vi "Spawn placeholder.vi"(11 "TEMPLATE Actor in":refnum<class "TEMPLATE Actor.lvclass">) -> (0 "Error out":errorcluster, 3 "TEMPLATE Actor out":refnum<class "TEMPLATE Actor.lvclass">)   [LabVIEW 2025, in "_Template.lvlib" / "Templates.lvlib" / "TEMPLATE Actor.lvlib" / "TEMPLATE Actor.lvclass"]
uses:
  TEMPLATE Actor.lvclass
  C:/git/jettl/src/jettl/jettl/Actor/Actor.lvclass
  Static Child UIDs.ctl
  TEMPLATE Actor.lvclass/TEMPLATE Actor.ctl
  C:/git/jettl/src/jettl Tools/_Template/Templates/TEMPLATE Actor/TEMPLATE Actor/TEMPLATE Actor.lvclass
  jettl/jettl/jettl.lvlib
  TEMPLATE Actor.lvlib
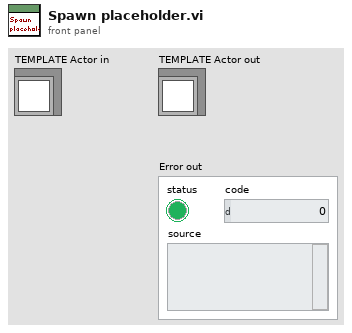
[diagram p1: front panel]
types:
  T1 = typedef "_Template.lvlib/Templates.lvlib/TEMPLATE Actor.lvlib/TEMPLATE Actor.lvclass/Static Child UIDs.ctl" = enum16{"placeholder"}
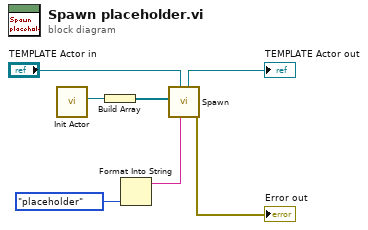
[diagram p0: block diagram]
diagram:
  n1 = call "Init Actor.vi"() -> ("Actor"=w3:refnum<class "Actor.lvclass">)  [unwired: 11 in]
  n2 = Build Array(w3) -> (w2:refnum<class "Actor.lvclass">[])
  n3 = Format Into String(Static_Child_UIDs."placeholder" ("Static Child UIDs")) -> (resulting string=w1:string)  [unwired: 3 in, 1 out]
  n4 = call "Spawn.vi"("UID"=w1, "Actor in"="TEMPLATE Actor in", "Local Layers"=w2) -> ("Error out"=→"Error out":errorcluster, "Actor out"=→"TEMPLATE Actor out":refnum<class "TEMPLATE Actor.lvclass">)  [unwired: 7 in]
